vi "MathOptim-Sigmoid Full Parameter Vector.vi"(0 "Y":dbl[](array[numeric]), 5 "X":dbl[](array[numeric]), 7 "a":dbl[](array[numeric])) -> (8 "Parameters":dbl[](array[numeric]))   [LabVIEW 2020]
doc: "This template is the starting point for creating a model function to be passed to the Nonlinear Curve Fit.vi."
uses:
  <vilib>/Analysis/7linalg.llb/Solve Linear Equations (single right hand).vi
  <vilib>/Analysis/baseanly.llb/Solve Linear Equations By Cholesky.vi
  <vilib>/Analysis/baseanly.llb/Real Matrix to Compact Array.vi
  <vilib>/Analysis/baseanly.llb/Real Compact Tri-Matrix Linear Eqs.vi
  <vilib>/Analysis/7linalg.llb/Solve Linear Eqs (General).vi
  <vilib>/Analysis/7linalg.llb/Solve Linear Eqs (Gen, single right hand).vi
  <vilib>/Analysis/NI_AALPro.lvlib
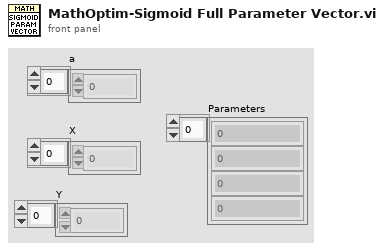
[diagram p1: front panel]
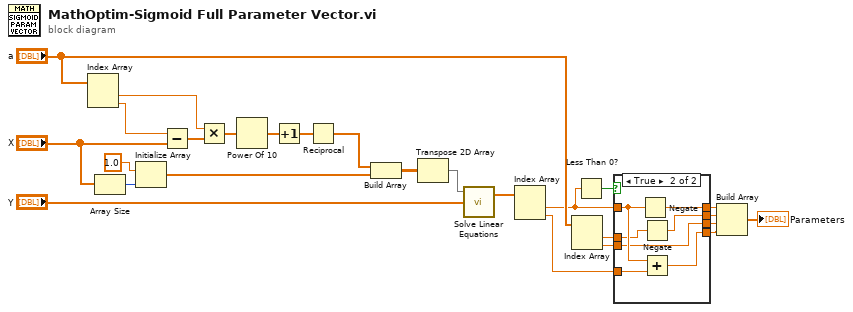
[diagram p0: block diagram]
diagram:
  n1 = Index Array(array="a") -> (element #1=w12:dbl, element #2=w15:dbl)  [unwired: 2 in]
  n2 = Array Size(array="X") -> (size(s)=w26:i32)
  n3 = Initialize Array(1.0, w26) -> (w24:dbl[])
  n4 = Subtract(x=w15, y="X") -> (x-y=w13:dbl[])
  n5 = Multiply(x=w12, y=w13) -> (x*y=w20:dbl[])
  n6 = Power Of 10(x=w20) -> (10^x=w11:dbl[])
  n7 = Increment(x=w11) -> (x+1=w19:dbl[])
  n8 = Reciprocal(x=w19) -> (1/x=w18:dbl[])
  n9 = Build Array(w18, w24) -> (w23:dbl[][])
  n10 = Transpose 2D Array(2D array=w23) -> (transposed array=w21:dbl[][])
  n11 = call-poly <vilib>:"Solve Linear Equations.vi"("Known Vector"="Y", "Input Matrix"=w21) -> ("Solution Vector"=w22:dbl[])  [unwired: 1 in, 1 out]
  n12 = Index Array(array=w22) -> (element #1=w1:dbl, element #2=w7:dbl)  [unwired: 2 in]
  n13 = Index Array(array="a") -> (element #1=w8:dbl, element #2=w6:dbl)  [unwired: 2 in]
  n14 = Less Than 0?(x=w1) -> (x < 0?=w2:bool)
  n15 = case shown="True" w2 {
    tunnel: w1 -> [w30 w35]
    tunnel: [w30 w34] -> w9
    tunnel: [w29 w31] -> w5
    tunnel: w8 -> [w29 w32]
    tunnel: w7 -> [w27 w37]
    tunnel: w6 -> [w28 w33]
    tunnel: [w28 w33] -> w4
    tunnel: [w27 w36] -> w3
    frame False {
    }
    frame True {
      n16 = Negate(x=w35) -> (-x=w34:dbl)
      n17 = Negate(x=w32) -> (-x=w31:dbl)
      n18 = Add(x=w35, y=w37) -> (x+y=w36:dbl)
    }
  }
  n19 = Build Array(w9, w5, w4, w3) -> (→"Parameters":dbl[])
